vi "内泄漏.vi"(8 "error in (no error)":errorcluster caption="错误输入（无错误）", 11 "信号数据":dbl[][](array[numeric])) -> (0 "error out":errorcluster caption="错误输出")   [LabVIEW 2015, in "Logging.lvlib"]
uses:
  Logging.lvlib
panel:
  out "右侧流量":dbl
  out "左侧流量":dbl
  in  "取消按钮":bool
  in  "确定按钮":bool
  # "内泄漏测量结果"
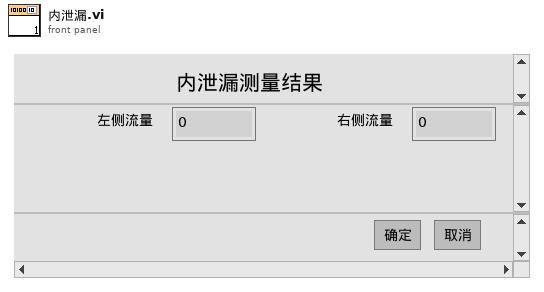
[diagram p1: front panel]
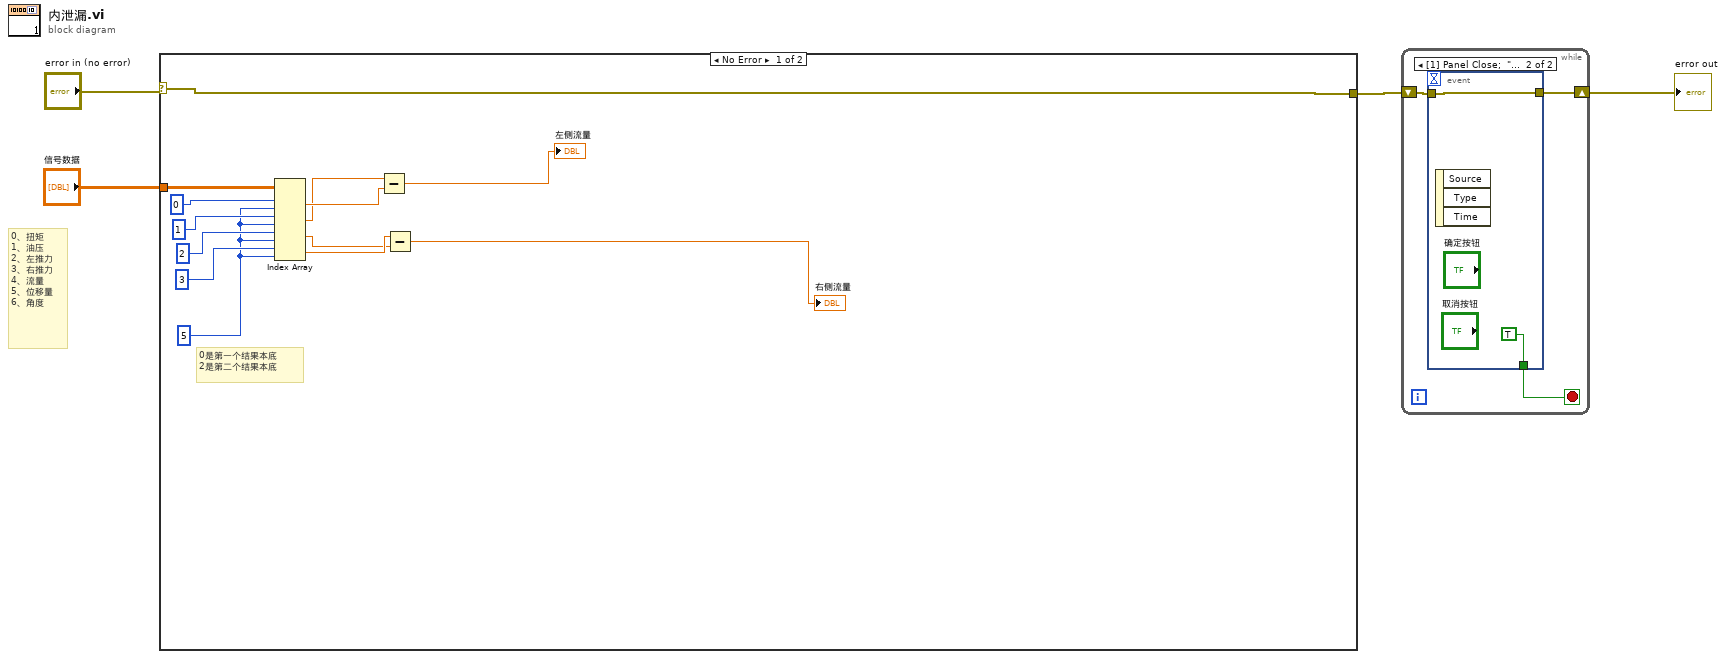
[diagram p0: block diagram]
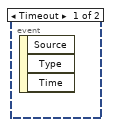
[diagram p2: hidden frame]
diagram:
  # "0、扭矩\n1、油压\n2、左推力\n3、右推力\n4、流量\n5、位移量\n6、角度"
  n1 = case shown="No Error" "error in (no error)" {
    selector: "error in (no error)" -> [w16 w18]
    tunnel: "信号数据" -> [w17 _]
    tunnel: [w16 w18] -> w1
    frame No Error {
      w8 = 5 ("禁用的索引 (列)")
      # "0是第一个结果本底\n2是第二个结果本底"
      n2 = Index Array(array=w17, index (row) #1=0 ("disabled index (row)"), index (col) #1=w8, index (row) #2=1 ("disabled index (row)"), index (col) #2=w8, index (row) #3=2 ("index (row)"), index (col) #3=w8, index (row) #4=3 ("index (row)"), index (col) #4=w8) -> (element #1=w11:dbl, element #2=w10:dbl, element #3=w6:dbl, element #4=w7:dbl)
      n3 = Subtract(x=w10, y=w11) -> (x-y=→"左侧流量":dbl)
      n4 = Subtract(x=w7, y=w6) -> (x-y=→"右侧流量":dbl)
    }
    frame Error {
    }
  }
  n5 = while {
    shift-right: [w21] -> w2
    shift-left: w1 -> [w20]
    stop <- w19 stop-if-true
    n6 = event shown="[1] Panel Close;  \"确定按钮\", \"取消按钮\": Value Change" {
      selector: _ -> [_ _]
      dyn-events: _ -> [_ _]
      timeout: _ -> [_ _]
      tunnel: [_ w23] -> w21
      tunnel: w20 -> [_ w23]
      tunnel: [_ TRUE] -> w19
      event Timeout {
        n7 = event-data() -> ()  [unwired: 1 in, 3 out]
      }
      event Panel Close; "确定按钮", "取消按钮": Value Change {
        n8 = event-data() -> ()  [unwired: 1 in, 3 out]
      }
    }
  }
  "error out" <- w2
